vi "Data Server.vi"() -> ()   [LabVIEW 2010]
doc: "Sends a specified waveform through a TCP port. The VI first listens for a connection and, once established, sends the number of bytes to be sent followed by the data. After the data is sent, the VI waits for an 'all received' signal from the client and then breaks the connection.\n\n<B>Note:</B> Requires the Data Client.vi located in the same library as this VI."
uses:
  3.0 Flow Control/3.0 List of Loops.ctl
  3.0-Global.vi
panel:
  in  "Port":u16=33483 min=1025 step=1
  # "Instructions:\n1. Open the Data Client.vi\n2. Run This VI first.\n3. Run the Data Client.vi Second.\n4. Adjust the # of Points Function, and Noise Level controls.\n5. Observe the Chart on the Data Client.vi.\n6. Stop This VI. The Data Client.vi will time out and stop."
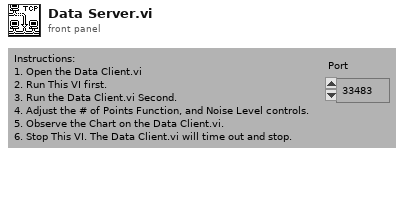
[diagram p1: front panel]
types:
  T1 = typedef "3.0 List of Loops.ctl" = enum16{"3.0 State Update", "3.0 GUI", "3.1 Act", "3.1 4.7.1 Act UDP", "3.1 Joystick", "3.2 Where", "3.2 4.7.2 Where UDP", "3.3 What", "3.3 4.7.3 What UDP", "3.4 How", "3.4 4.7.4 How UDP", "3.5 Limbic", "3.8 TCP", "3.6 Cerebellum"}
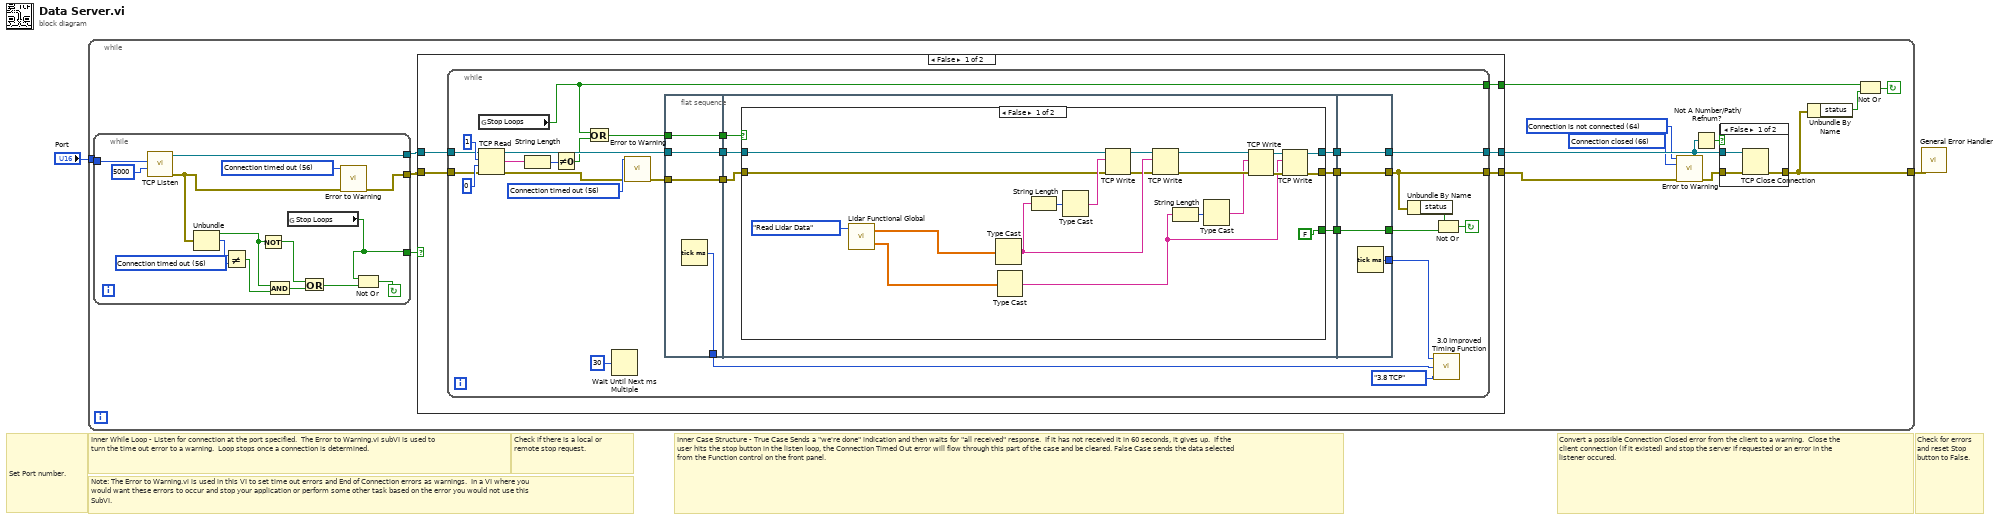
[diagram p0: block diagram]
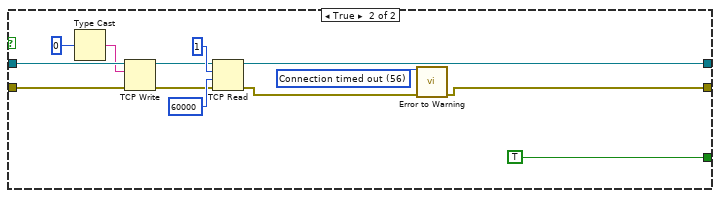
[diagram p2: hidden frame]
diagram:
  # "Check for errors\nand reset Stop \nbutton to False."
  # "Inner Case Structure - True Case Sends a \"we're done\" indication and then waits for \"all received\" response.  If it has not received it in 60 seconds, it gives up.  If the user hits the stop button in the listen loop, the Connection Timed Out error will flow through this part of the case and be cleared. False Case sends the data selected from the Function control on the front panel."
  # "Check if there is a local or remote stop request."
  # "Set Port number."
  # "Inner While Loop - Listen for connection at the port specified.  The Error to Warning.vi subVI is used to turn the time out error to a warning.  Loop stops once a connection is determined."
  # "Note: The Error to Warning.vi is used in this VI to set time out errors and End of Connection errors as warnings.  In a VI where you would want these errors to occur and stop your application or perform some other task based on the error you would not use this SubVI."
  # "Convert a possible Connection Closed error from the client to a warning.  Close the client connection (if it existed) and stop the server if requested or an error in the listener occured."
  n1 = while {
    tunnel: [w9] -> w1
    tunnel: "Port" -> [w15]
    stop <- w16 continue-if-true
    w5 = 66 items=["No Error", "Argument Error", "Memory Full", "Out of Zone", "End of File", "File Already Open", "Generic File IO Error", "File Not Found", "File Permission Error", "Disk Full", "Duplicate Path", "Too Many Files Open", "Not Enabled", "Resource File Not Found", "Cannot Add Resource", "Resource Not Found", "Image Not Found", "Image Memory Error", "Pen Does Not Exist", "Config Bad Type", "Config Token Not Found", "Config Parse Error", "Config Memory Error", "Bad External Code Format", "Bad External Code Offset", "External Code Not Present", "Null Window", "Destroy Window Mixup", "Null Menu", "Print Aborted", "Bad Print Record", "Print Driver Error", "Windows Error During Print", "Memory Error During Print", "Print Dialog Error", "Generic Print Error", "Invalid Device Refnum", "Device Not Found", "Device Parameter Error", "Device Unit Error", "Can't Open Device", "Device Call Aborted", "Generic Error", "Cancelled By User", "Object ID Too Low", "Object ID Too High", "Object Not In Heap", "Unknown Heap", "Bad DefProc ID", "DefProc Not In Table", "Message Out Of Range", "Null Method", "Unknown Message", "Manager Call Not Supported", "Bad address", "Connection In progress", "Connection timed out", "Connection is already in progress", "Network attribute not supported", "Network error", "Address in use", "System out of memory", "Connection aborted", "Connection refused", "Connection is not connected", "Connection is already connected", "Connection closed", "Initialize error (interapplication manager)", "Bad occurrence", "Wait on unbound occurrence handler", "Occurrence queue overflow", "Bad path", "Semaphore not signaled", "Unrecognized type (interapplication manager)"] ("2nd Error to Convert")
    w6 = 64 items=["No Error", "Argument Error", "Memory Full", "Out of Zone", "End of File", "File Already Open", "Generic File IO Error", "File Not Found", "File Permission Error", "Disk Full", "Duplicate Path", "Too Many Files Open", "Not Enabled", "Resource File Not Found", "Cannot Add Resource", "Resource Not Found", "Image Not Found", "Image Memory Error", "Pen Does Not Exist", "Config Bad Type", "Config Token Not Found", "Config Parse Error", "Config Memory Error", "Bad External Code Format", "Bad External Code Offset", "External Code Not Present", "Null Window", "Destroy Window Mixup", "Null Menu", "Print Aborted", "Bad Print Record", "Print Driver Error", "Windows Error During Print", "Memory Error During Print", "Print Dialog Error", "Generic Print Error", "Invalid Device Refnum", "Device Not Found", "Device Parameter Error", "Device Unit Error", "Can't Open Device", "Device Call Aborted", "Generic Error", "Cancelled By User", "Object ID Too Low", "Object ID Too High", "Object Not In Heap", "Unknown Heap", "Bad DefProc ID", "DefProc Not In Table", "Message Out Of Range", "Null Method", "Unknown Message", "Manager Call Not Supported", "Bad address", "Connection In progress", "Connection timed out", "Connection is already in progress", "Network attribute not supported", "Network error", "Address in use", "System out of memory", "Connection aborted", "Connection refused", "Connection is not connected", "Connection is already connected", "Connection closed", "Initialize error (interapplication manager)", "Bad occurrence", "Wait on unbound occurrence handler", "Occurrence queue overflow", "Bad path", "Semaphore not signaled", "Unrecognized type (interapplication manager)"] ("1st Error to Convert")
    n2 = while {
      tunnel: [w17] -> w12
      tunnel: [w26] -> w13
      tunnel: [w30] -> w14
      tunnel: w15 -> [w31]
      stop <- w28 continue-if-true
      w24 = 56 items=["No Error", "Argument Error", "Memory Full", "Out of Zone", "End of File", "File Already Open", "Generic File IO Error", "File Not Found", "File Permission Error", "Disk Full", "Duplicate Path", "Too Many Files Open", "Not Enabled", "Resource File Not Found", "Cannot Add Resource", "Resource Not Found", "Image Not Found", "Image Memory Error", "Pen Does Not Exist", "Config Bad Type", "Config Token Not Found", "Config Parse Error", "Config Memory Error", "Bad External Code Format", "Bad External Code Offset", "External Code Not Present", "Null Window", "Destroy Window Mixup", "Null Menu", "Print Aborted", "Bad Print Record", "Print Driver Error", "Windows Error During Print", "Memory Error During Print", "Print Dialog Error", "Generic Print Error", "Invalid Device Refnum", "Device Not Found", "Device Parameter Error", "Device Unit Error", "Can't Open Device", "Device Call Aborted", "Generic Error", "Cancelled By User", "Object ID Too Low", "Object ID Too High", "Object Not In Heap", "Unknown Heap", "Bad DefProc ID", "DefProc Not In Table", "Message Out Of Range", "Null Method", "Unknown Message", "Manager Call Not Supported", "Bad address", "Connection In progress", "Connection timed out", "Connection is already in progress", "Network attribute not supported", "Network error", "Address in use", "System out of memory", "Connection aborted", "Connection refused", "Connection is not connected", "Connection is already connected", "Connection closed", "Initialize error (interapplication manager)", "Bad occurrence", "Wait on unbound occurrence handler", "Occurrence queue overflow", "Bad path", "Semaphore not signaled", "Unrecognized type (interapplication manager)"] ("1st Error to Convert")
      w25 = 56 items=["No Error", "Argument Error", "Memory Full", "Out of Zone", "End of File", "File Already Open", "Generic File IO Error", "File Not Found", "File Permission Error", "Disk Full", "Duplicate Path", "Too Many Files Open", "Not Enabled", "Resource File Not Found", "Cannot Add Resource", "Resource Not Found", "Image Not Found", "Image Memory Error", "Pen Does Not Exist", "Config Bad Type", "Config Token Not Found", "Config Parse Error", "Config Memory Error", "Bad External Code Format", "Bad External Code Offset", "External Code Not Present", "Null Window", "Destroy Window Mixup", "Null Menu", "Print Aborted", "Bad Print Record", "Print Driver Error", "Windows Error During Print", "Memory Error During Print", "Print Dialog Error", "Generic Print Error", "Invalid Device Refnum", "Device Not Found", "Device Parameter Error", "Device Unit Error", "Can't Open Device", "Device Call Aborted", "Generic Error", "Cancelled By User", "Object ID Too Low", "Object ID Too High", "Object Not In Heap", "Unknown Heap", "Bad DefProc ID", "DefProc Not In Table", "Message Out Of Range", "Null Method", "Unknown Message", "Manager Call Not Supported", "Bad address", "Connection In progress", "Connection timed out", "Connection is already in progress", "Network attribute not supported", "Network error", "Address in use", "System out of memory", "Connection aborted", "Connection refused", "Connection is not connected", "Connection is already connected", "Connection closed", "Initialize error (interapplication manager)", "Bad occurrence", "Wait on unbound occurrence handler", "Occurrence queue overflow", "Bad path", "Semaphore not signaled", "Unrecognized type (interapplication manager)"] ("1st Error to Convert")
      n3 = call <vilib>:"TCP Listen.vi"("timeout ms (wait forever: -1)"=5000, "port"=w31) -> ("error out"=w27:errorcluster, "connection ID"=w30:refnum<k5>)  [unwired: 6 in, 2 out]
      n4 = Unbundle(w27) -> ("status"=w22:bool, "code"=w23:i32)  [unwired: 1 out]
      n5 = Not Equal?(x=w23, y=w24) -> (x != y?=w21:bool)
      n6 = Not(x=w22) -> (.not. x?=w20:bool)
      n7 = And(x=w22, y=w21) -> (x .and. y?=w19:bool)
      n8 = global read "3.0-Global.vi" "Stop Loops"() -> (w17:bool)
      n9 = Or(x=w20, y=w19) -> (x .or. y?=w18:bool)
      n10 = call <vilib>:"Error to Warning.vi"("1st Error to Convert"=w25, "error in"=w27) -> ("warning out"=w26:errorcluster)  [unwired: 13 in]
      n11 = Not Or(1:w18, 2:w17) -> (0:w28:bool)
    }
    n12 = case shown="False" w12 {
      selector: w12 -> [_ w112]
      tunnel: [w36 w113] -> w4
      tunnel: w14 -> [w35 w114]
      tunnel: w13 -> [w34 w113]
      tunnel: [w33 w114] -> w11
      tunnel: [w32 w112] -> w7
      frame False {
        n13 = while {
          tunnel: [w47] -> w32
          tunnel: w34 -> [w61]
          tunnel: [w52] -> w36
          tunnel: [w57] -> w33
          tunnel: w35 -> [w60]
          stop <- w64 continue-if-true
          w50 = 56 items=["No Error", "Argument Error", "Memory Full", "Out of Zone", "End of File", "File Already Open", "Generic File IO Error", "File Not Found", "File Permission Error", "Disk Full", "Duplicate Path", "Too Many Files Open", "Not Enabled", "Resource File Not Found", "Cannot Add Resource", "Resource Not Found", "Image Not Found", "Image Memory Error", "Pen Does Not Exist", "Config Bad Type", "Config Token Not Found", "Config Parse Error", "Config Memory Error", "Bad External Code Format", "Bad External Code Offset", "External Code Not Present", "Null Window", "Destroy Window Mixup", "Null Menu", "Print Aborted", "Bad Print Record", "Print Driver Error", "Windows Error During Print", "Memory Error During Print", "Print Dialog Error", "Generic Print Error", "Invalid Device Refnum", "Device Not Found", "Device Parameter Error", "Device Unit Error", "Can't Open Device", "Device Call Aborted", "Generic Error", "Cancelled By User", "Object ID Too Low", "Object ID Too High", "Object Not In Heap", "Unknown Heap", "Bad DefProc ID", "DefProc Not In Table", "Message Out Of Range", "Null Method", "Unknown Message", "Manager Call Not Supported", "Bad address", "Connection In progress", "Connection timed out", "Connection is already in progress", "Network attribute not supported", "Network error", "Address in use", "System out of memory", "Connection aborted", "Connection refused", "Connection is not connected", "Connection is already connected", "Connection closed", "Initialize error (interapplication manager)", "Bad occurrence", "Wait on unbound occurrence handler", "Occurrence queue overflow", "Bad path", "Semaphore not signaled", "Unrecognized type (interapplication manager)"] ("1st Error to Convert")
          n14 = global read "3.0-Global.vi" "Stop Loops"() -> (w47:bool)
          n15 = TCP Read(connection ID=w60, bytes to read=1, error in (no error)=w61, 9:0) -> (connection ID out=w58:refnum<k5>, data out=w59:string, error out=w49:errorcluster)  [unwired: 1 in]
          n16 = String Length(string=w59) -> (length=w55:i32)
          n17 = Not Equal To 0?(x=w55) -> (x != 0?=w54:bool)
          n18 = Or(x=w47, y=w54) -> (x .or. y?=w53:bool)
          n19 = Wait Until Next ms Multiple(millisecond multiple=u32 30 ("milliseconds to wait")) -> ()  [unwired: 1 out]
          n20 = call <vilib>:"Error to Warning.vi"("1st Error to Convert"=w50, "error in"=w49) -> ("warning out"=w48:errorcluster)  [unwired: 13 in]
          n21 = flat-sequence {
            tunnel: w48 -> [w66]
            tunnel: w53 -> [w67]
            tunnel: w58 -> [w68]
            tunnel: [w68] -> w43
            tunnel: [w67] -> w42
            tunnel: [w66] -> w41
            tunnel: [w65] -> w38
            tunnel: [w73] -> w46
            tunnel: [w72] -> w45
            tunnel: [w70] -> w44
            tunnel: w43 -> [w74]
            tunnel: w42 -> [w71]
            tunnel: w41 -> [w69]
            tunnel: [w109] -> w52
            tunnel: [w110] -> w56
            tunnel: [w111] -> w57
            tunnel: w46 -> [w111]
            tunnel: w45 -> [w110]
            tunnel: w44 -> [w109]
            tunnel: [w108] -> w39
            frame #0 {
              n22 = Tick Count (ms)() -> (millisecond timer value=w65:u32)
            }
            frame #1 {
              n23 = case shown="False" w71 {
                tunnel: w69 -> [w89 w103]
                tunnel: w74 -> [w88 w101]
                tunnel: [w76 w105] -> w73
                tunnel: [w75 w96] -> w70
                tunnel: [FALSE TRUE] -> w72
                frame False {
                  n24 = call "Lidar Functional Global.vi"("Lidar Action"=enum16{"Set Lidar Data", "Read Lidar Data"}."Read Lidar Data") -> ("Lidar Angle Data Out (Degrees)"=w82:sgl[], "Lidar Magnitude Data Out (mm)"=w85:sgl[])  [unwired: 2 in]
                  n25 = Type Cast(x=w85) -> (*(type *) &x=w94:string)  [unwired: 1 in]
                  n26 = Type Cast(x=w82) -> (*(type *) &x=w77:string)  [unwired: 1 in]
                  n27 = String Length(string=w94) -> (length=w92:i32)
                  n28 = Type Cast(x=w92) -> (*(type *) &x=w93:string)  [unwired: 1 in]
                  n29 = TCP Write(connection ID=w88, data in=w93, error in (no error)=w89) -> (connection ID out=w90:refnum<k5>, error out=w91:errorcluster)  [unwired: 1 in, 1 out]
                  n30 = TCP Write(connection ID=w90, data in=w94, error in (no error)=w91) -> (connection ID out=w83:refnum<k5>, error out=w84:errorcluster)  [unwired: 1 in, 1 out]
                  n31 = String Length(string=w77) -> (length=w81:i32)
                  n32 = Type Cast(x=w81) -> (*(type *) &x=w80:string)  [unwired: 1 in]
                  n33 = TCP Write(connection ID=w83, data in=w80, error in (no error)=w84) -> (connection ID out=w78:refnum<k5>, error out=w79:errorcluster)  [unwired: 1 in, 1 out]
                  n34 = TCP Write(connection ID=w78, data in=w77, error in (no error)=w79) -> (connection ID out=w76:refnum<k5>, error out=w75:errorcluster)  [unwired: 1 in, 1 out]
                }
                frame True {
                  w95 = 56 items=["No Error", "Argument Error", "Memory Full", "Out of Zone", "End of File", "File Already Open", "Generic File IO Error", "File Not Found", "File Permission Error", "Disk Full", "Duplicate Path", "Too Many Files Open", "Not Enabled", "Resource File Not Found", "Cannot Add Resource", "Resource Not Found", "Image Not Found", "Image Memory Error", "Pen Does Not Exist", "Config Bad Type", "Config Token Not Found", "Config Parse Error", "Config Memory Error", "Bad External Code Format", "Bad External Code Offset", "External Code Not Present", "Null Window", "Destroy Window Mixup", "Null Menu", "Print Aborted", "Bad Print Record", "Print Driver Error", "Windows Error During Print", "Memory Error During Print", "Print Dialog Error", "Generic Print Error", "Invalid Device Refnum", "Device Not Found", "Device Parameter Error", "Device Unit Error", "Can't Open Device", "Device Call Aborted", "Generic Error", "Cancelled By User", "Object ID Too Low", "Object ID Too High", "Object Not In Heap", "Unknown Heap", "Bad DefProc ID", "DefProc Not In Table", "Message Out Of Range", "Null Method", "Unknown Message", "Manager Call Not Supported", "Bad address", "Connection In progress", "Connection timed out", "Connection is already in progress", "Network attribute not supported", "Network error", "Address in use", "System out of memory", "Connection aborted", "Connection refused", "Connection is not connected", "Connection is already connected", "Connection closed", "Initialize error (interapplication manager)", "Bad occurrence", "Wait on unbound occurrence handler", "Occurrence queue overflow", "Bad path", "Semaphore not signaled", "Unrecognized type (interapplication manager)"] ("1st Error to Convert")
                  n35 = Type Cast(x=0) -> (*(type *) &x=w98:string)  [unwired: 1 in]
                  n36 = TCP Write(connection ID=w101, data in=w98, error in (no error)=w103) -> (connection ID out=w100:refnum<k5>, error out=w102:errorcluster)  [unwired: 1 in, 1 out]
                  n37 = TCP Read(connection ID=w100, bytes to read=1, error in (no error)=w102, 9:60000) -> (connection ID out=w105:refnum<k5>, error out=w97:errorcluster)  [unwired: 1 in, 1 out]
                  n38 = call <vilib>:"Error to Warning.vi"("1st Error to Convert"=w95, "error in"=w97) -> ("warning out"=w96:errorcluster)  [unwired: 13 in]
                }
              }
            }
            frame #2 {
              n39 = Tick Count (ms)() -> (millisecond timer value=w108:u32)
            }
          }
          n40 = Unbundle By Name(w52) -> ("status"=w51:bool)
          n41 = call "3.0 Improved Timing Function.vi"("Loop"=3.0_List_of_Loops."3.8 TCP", "Start"=w38, "End"=w39) -> ()  [unwired: 1 in]
          n42 = Not Or(1:w56, 2:w51) -> (0:w64:bool)
        }
      }
      frame True {
      }
    }
    n43 = call <vilib>:"Error to Warning.vi"("1st Error to Convert"=w6, "2nd Error to Convert"=w5, "error in"=w4) -> ("warning out"=w3:errorcluster)  [unwired: 12 in]
    n44 = Not A Number/Path/Refnum?(number/path/refnum=w11) -> (NaN/Path/Refnum?=w10:bool)
    n45 = case shown="False" w10 {
      tunnel: w3 -> [w117 w118]
      tunnel: w11 -> [w116 _]
      tunnel: [w115 w118] -> w9
      frame False {
        n46 = TCP Close Connection(connection ID=w116, error in (no error)=w117) -> (error out=w115:errorcluster)  [unwired: 1 in, 1 out]
      }
      frame True {
      }
    }
    n47 = Unbundle By Name(w9) -> ("status"=w8:bool)
    n48 = Not Or(1:w8, 2:w7) -> (0:w16:bool)
  }
  n49 = call <vilib>:"General Error Handler.vi"("error in (no error)"=w1) -> ()  [unwired: 10 in, 5 out]
